vi "Read Mods.vi"(8 "error in (no error)":errorcluster, 11 "ListboxDoubleClickMsg in":refnum<class "ListboxDoubleClickMsg.lvclass">) -> (0 "error out":errorcluster, 2 "Mods":cluster{"Double Click":bool, "Menu Key":bool}, 3 "ListboxDoubleClickMsg out":refnum<class "ListboxDoubleClickMsg.lvclass">)   [LabVIEW 2019, in "ActorEvents.lvlib" / "ListboxDoubleClickMsg.lvclass"]
uses:
  <vilib>/gpm_packages/@cs/mva-viewable/Source/ActorEvents/IEventAggregator Messages/ListboxDoubleClickMsg/ListboxDoubleClickMsg.lvclass
  <vilib>/gpm_packages/@cs/mva-viewable/Source/ActorEvents/IEventAggregator Messages/ListboxDoubleClickMsg/ListboxDoubleClickMsg.lvclass/ListboxDoubleClickMsg.ctl
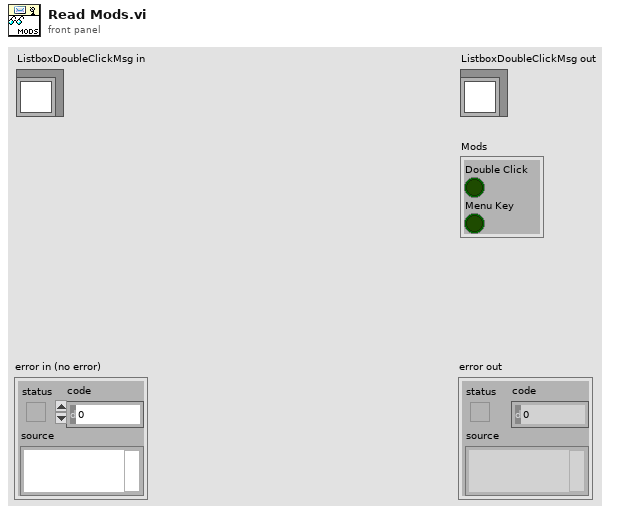
[diagram p1: front panel]
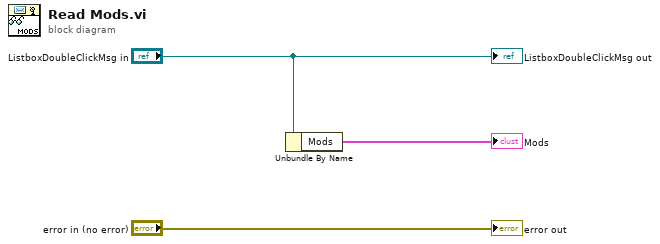
[diagram p0: block diagram]
diagram:
  n1 = Unbundle By Name("ListboxDoubleClickMsg in") -> ("Mods"=→"Mods":cluster{"Double Click":bool, "Menu Key":bool})
  "error out" <- "error in (no error)"
  "ListboxDoubleClickMsg out" <- "ListboxDoubleClickMsg in"
